vi "CAN Start Schedule.vi"(6 "OrderSend":u8, 7 "TimePrecMs":u8, 9 "MsgTabIndex":u8, 10 "CANIndex":u8, 11 "DevHandle":i32) -> (3 "function return":i32)   [LabVIEW 2010, in "usb2can.lvlib"]
doc: "int WINAPI CAN_StartSchedule(int DevHandle, unsigned char CANIndex, unsigned char MsgTabIndex,unsigned char TimePrecMs,unsigned char OrderSend);"
uses:
  usb2can.lvlib
  USB2XXX/trunk/USB2XXX/USB2XXX/vs2019/Release/USB2XXX.dll
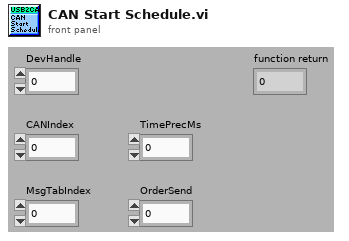
[diagram p1: front panel]
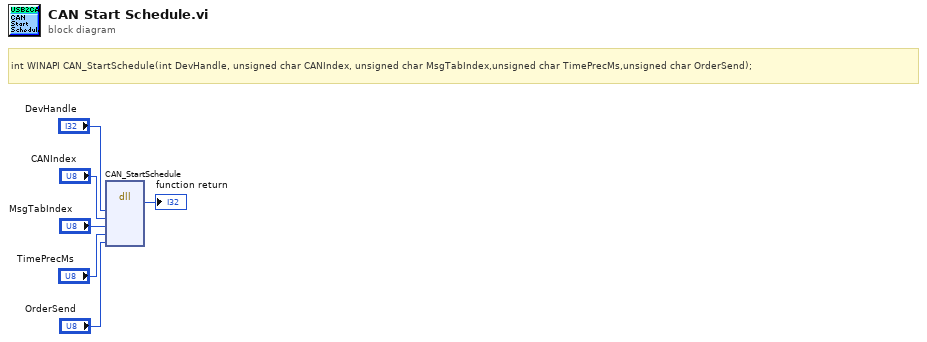
[diagram p0: block diagram]
diagram:
  # "int WINAPI CAN_StartSchedule(int DevHandle, unsigned char CANIndex, unsigned char MsgTabIndex,unsigned char TimePrecMs,unsigned char OrderSend);"
  n1 = dll-call lib="E:/Projects/USB2XXX/trunk/USB2XXX/USB2XXX/vs2019/Release/USB2XXX.*" fn="CAN_StartSchedule"("DevHandle"="DevHandle", "CANIndex"="CANIndex", "MsgTabIndex"="MsgTabIndex", "TimePrecMs"="TimePrecMs", "OrderSend"="OrderSend") -> (→"function return":i32)  [unwired: 8 in, 2 out]
